vi "Collimation.vi"(0 "Motion Controller in":refnum<class "Motion Controller.lvclass">, 1 "Beam Profiler in":refnum<class "Beam Profiler.lvclass">, 3 "Peak responsivity [%,0-100]":dbl, 4 "Knife Edge in":T1={"X"=nan, "Y"=nan}, 5 "Error in":errorcluster, 6 "Step":dbl[unit], 7 "Start Position":dbl[unit], 9 "Stop Collimation Position":dbl[unit], 10 "Cancel?":bool) -> (11 "Stop positon":dbl[unit], 12 "Cancel Test":bool, 13 "数组":dbl[][](array[numeric]), 14 "Motion Controller out":refnum<class "Motion Controller.lvclass">, 15 "Beam Profiler out":refnum<class "Beam Profiler.lvclass">, 17 "Peak responsivity [%,0-100] out":dbl, 18 "Knife Edge out":T1={"X"=nan, "Y"=nan}, 19 "Error out":errorcluster)   [LabVIEW 2018]
uses:
  <instrlib>/nLight Instruments/Motion Controller/Motion Controller.lvclass
  <instrlib>/nLight Instruments/Beam Profiler/Beam profiler XY distance value pair.ctl
  <instrlib>/nLight Instruments/Beam Profiler/Beam Profiler.lvclass
  <instrlib>/nLight Instruments/Motion Controller/Axis index.ctl
  <instrlib>/nLight Instruments/Motion Controller/Move axis absolute distance units.vi
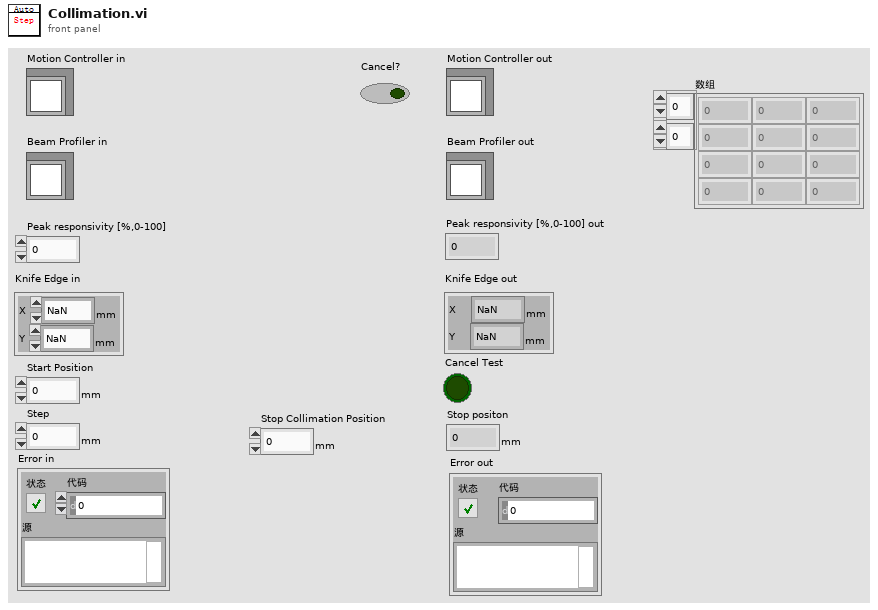
[diagram p1: front panel]
types:
  T1 = typedef "Beam Profiler.lvclass/Beam profiler XY distance value pair.ctl" = cluster{"X":dbl[unit], "Y":dbl[unit]}
  T2 = typedef "Motion Controller.lvclass/Axis index.ctl" = i32
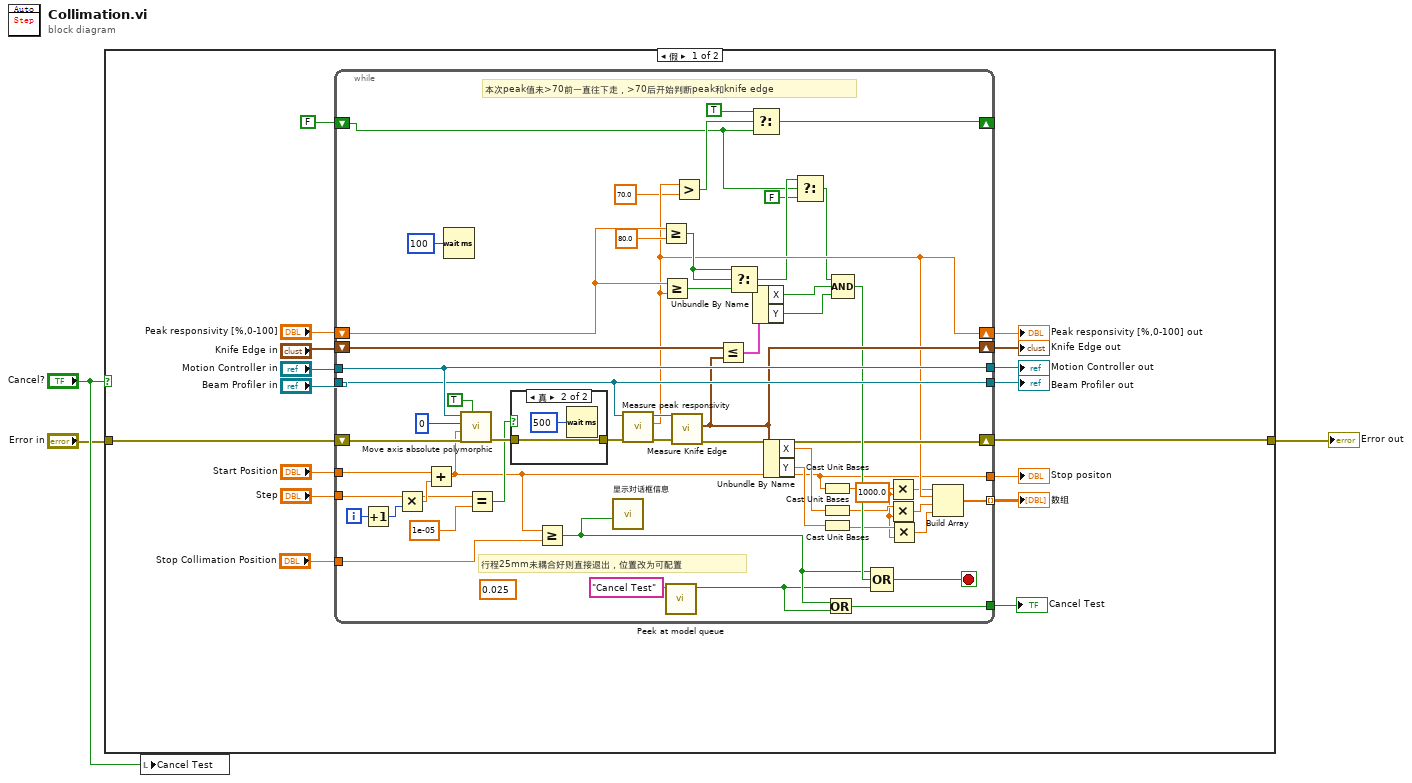
[diagram p0: block diagram]
diagram:
  n1 = case shown="假" "Cancel?" {
    tunnel: "Error in" -> [w19 w78]
    tunnel: [w8 w78] -> w3
    frame False {
      n2 = while {
        shift-right: [w46] -> w17
        shift-left: "Peak responsivity [%,0-100]" -> [w51]
        shift-right: [w53] -> w15
        shift-left: "Knife Edge in" -> [w69]
        tunnel: "Beam Profiler in" -> [w66]
        tunnel: "Motion Controller in" -> [w67]
        shift-right: [w49] -> w8
        shift-left: w19 -> [w74]
        tunnel: "Step" -> [w32]
        tunnel: [w67] -> w9
        tunnel: [w66] -> w4
        tunnel: [w22] -> w14
        tunnel: "Start Position" -> [w61]
        tunnel: [w25] -> w11
        tunnel: [w52] -> w10 mode=indexing
        shift-right: [w27] -> _
        shift-left: FALSE -> [w26]
        tunnel: "Stop Collimation Position" -> [w21]
        i -> [w58]
        stop <- w57 stop-if-true
        (unwired) dbl[unit] 0.025 ("y")
        w35 = 1000.0 ("y")
        # "行程25mm未耦合好则直接退出，位置改为可配置"
        # "本次peak值未>70前一直往下走，>70后开始判断peak和knife edge"
        n3 = Increment(x=w58) -> (x+1=w60:i32)
        n4 = Multiply(x=w32, y=w60) -> (x*y=w59:dbl[unit])
        n5 = Add(x=w61, y=w59) -> (x+y=w25:dbl[unit])
        n6 = Wait (ms)(milliseconds to wait=u32 100 ("等待时间（毫秒）")) -> ()  [unwired: 1 out]
        n7 = call-poly <instrlib>:"Move axis absolute polymorphic.vi"("Wait? (T)"=TRUE, "error in (no error)"=w74, "Move location"=w25, "Axis index"=T2 0, "Motion Controller in"=w67) -> ("error out"=w34:errorcluster)  [unwired: 5 in, 1 out]
        n8 = Equal?(x=w32, y=dbl[unit] 1e-05) -> (x = y?=w30:bool)
        n9 = case shown="真" w30 {
          tunnel: w34 -> [w75 w77]
          tunnel: [w75 w77] -> w33
          frame False {
          }
          frame True {
            n10 = Wait (ms)(milliseconds to wait=u32 500 ("等待时间（毫秒）")) -> ()  [unwired: 1 out]
          }
        }
        n11 = Greater Or Equal?(x=w25, y=w21) -> (x >= y?=w24:bool)
        n12 = call "显示对话框信息"("Enable"=w24) -> ()  [unwired: 9 in, 2 out]
        n13 = call-dynamic "Measure peak responsivity.vi"("error in (no error)"=w33, "Beam Profiler in"=w66) -> ("error out"=w71:errorcluster, "Peak responsivity [%,0-100]"=w46:dbl, "Beam Profiler out"=w70:refnum<class "Beam Profiler.lvclass">)  [unwired: 7 in]
        n14 = Greater Or Equal?(x=w51, y=80.0) -> (x >= y?=w55:bool)
        n15 = Greater Or Equal?(x=w51, y=w46) -> (x >= y?=w54:bool)
        n16 = call "Peek at model queue.vi"("Check for specific pending state (don't check)"="Cancel Test") -> ("Specific pending state found"=w23:bool)  [unwired: 7 in, 3 out]
        n17 = call-dynamic "Measure Knife Edge.vi"("error in (no error)"=w71, "Beam Profiler 输入"=w70) -> ("error out"=w49:errorcluster, "Knife Edge"=w53:T1)  [unwired: 7 in, 1 out]
        n18 = Greater?(x=w46, y=70.0) -> (0:w29:bool)
        n19 = Less Or Equal?(x=w69, y=w53) -> (x <= y?=w65:cluster{"X":bool, "Y":bool})
        n20 = Select(t=w55, s=w55, f=w54) -> (s? t:f=w44:bool)
        n21 = Select(t=TRUE, s=w29, f=w26) -> (s? t:f=w27:bool)
        n22 = Unbundle By Name(w65) -> ("X"=w64:bool, "Y"=w63:bool)
        n23 = Unbundle By Name(w53) -> ("X"=w48:dbl[unit], "Y"=w47:dbl[unit])
        n24 = Select(t=w44, s=w26, f=FALSE) -> (s? t:f=w42:bool)
        n25 = Cast Unit Bases(0:w25) -> (2:w41:dbl)  [unwired: 1 in]
        n26 = Cast Unit Bases(0:w48) -> (2:w38:dbl)  [unwired: 1 in]
        n27 = Cast Unit Bases(0:w47) -> (2:w36:dbl)  [unwired: 1 in]
        n28 = Or(x=w24, y=w23) -> (x .or. y?=w22:bool)
        n29 = Compound Arithmetic op=AND ("复合运算")(w42, w64, w63) -> (w50:bool)
        n30 = Compound Arithmetic op=OR ("复合运算")(w24, w50, w23) -> (w57:bool)
        n31 = Multiply(x=w41, y=w35) -> (x*y=w40:dbl)
        n32 = Multiply(x=w38, y=w35) -> (x*y=w39:dbl)
        n33 = Multiply(x=w36, y=w35) -> (x*y=w37:dbl)
        n34 = Build Array(w40, w46, w39, w37) -> (w52:dbl[])
      }
      "Peak responsivity [%,0-100] out" <- w17
      "Motion Controller out" <- w9
      "Knife Edge out" <- w15
      "Cancel Test" <- w14
      "Stop positon" <- w11
      "数组" <- w10
      "Beam Profiler out" <- w4
    }
    frame True {
    }
  }
  "Error out" <- w3
  n35 = local write "Cancel Test"("Cancel?") -> ()
